vi "waitStatusIdle.vi"(8 "error in (no error)":errorcluster, 11 "Instrument.LockinAPI in":refnum<class "Instrument.LockinAPI.lvclass">) -> (0 "error out":errorcluster, 3 "Instrument.LockinAPI out":refnum<class "Instrument.LockinAPI.lvclass">)   [LabVIEW 2019, in "Instrument.LockinAPI.lvclass"]
uses:
  Instrument.LockinAPI.lvclass
  Typedefs/LockinAPI.getState.states--enum.ctl
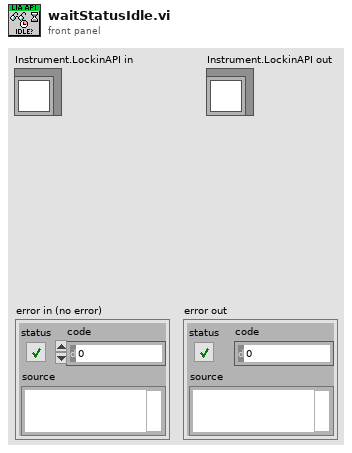
[diagram p1: front panel]
types:
  T1 = typedef "Instrument.LockinAPI.lvclass/LockinAPI.getState.states--enum.ctl" = enum16{"idle", "created", "started", "stopped", "sweeping"}
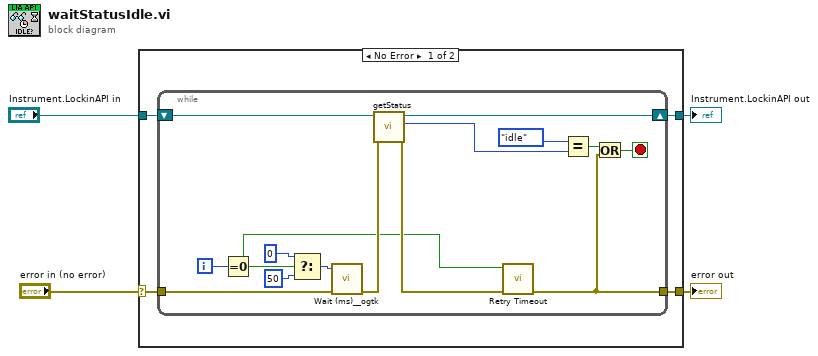
[diagram p0: block diagram]
diagram:
  n1 = case shown="No Error" "error in (no error)" {
    selector: "error in (no error)" -> [w5 w24]
    tunnel: [w8 w24] -> w4
    tunnel: [w7 w25] -> w3
    tunnel: "Instrument.LockinAPI in" -> [w6 w25]
    frame No Error {
      n2 = while {
        tunnel: w5 -> [w23]
        tunnel: [w13] -> w8
        shift-right: [w17] -> w7
        shift-left: w6 -> [w18]
        i -> [w11]
        stop <- w22 stop-if-true
        n3 = Equal To 0?(x=w11) -> (x = 0?=w10:bool)
        n4 = Select(t=u32 0, s=w10, f=u32 50 ("milliseconds to wait")) -> (s? t:f=w19:u32)
        n5 = call <userlib>:"Wait (ms)__ogtk.vi"("error in (no error)"=w23, "milliseconds to wait"=w19) -> ("error out"=w14:errorcluster)  [unwired: 8 in, 1 out]
        n6 = call-dynamic "getStatus.vi"("error in (no error)"=w14, "Instrument.LockinAPI in"=w18) -> ("error out"=w12:errorcluster, "state"=w16:T1, "Instrument.LockinAPI out"=w17:refnum<class "Instrument.LockinAPI.lvclass">)  [unwired: 7 in]
        n7 = call "Retry Timeout.vi"("error in (no error)"=w12, "reset"=w10) -> ("error out"=w13:errorcluster)  [unwired: 8 in, 1 out]
        n8 = Equal?(x=LockinAPI.getState.states--enum."idle" ("state"), y=w16) -> (x = y?=w15:bool)
        n9 = Or(x=w15, y=w13) -> (x .or. y?=w22:bool)
      }
    }
    frame Error {
    }
  }
  "error out" <- w4
  "Instrument.LockinAPI out" <- w3
